vi "SetMaxDrivingPower.vi"(9 "Reinit":bool, 10 "HMI to Control":T1, 11 "SensorInputData":T2) -> (2 "HMI to ControlOut":T1, 3 "SensorInputDataOut":T2, 4 "Done":bool=TRUE)   [LabVIEW 2015]
uses:
  Gensubs/Maximum Power Allowed.vi
  Typedefs/SensorInputData.ctl
  Typedefs/HMI_to_Control.ctl
panel:
  in  "arguments":string[](array[string])
  in  "dt":i32
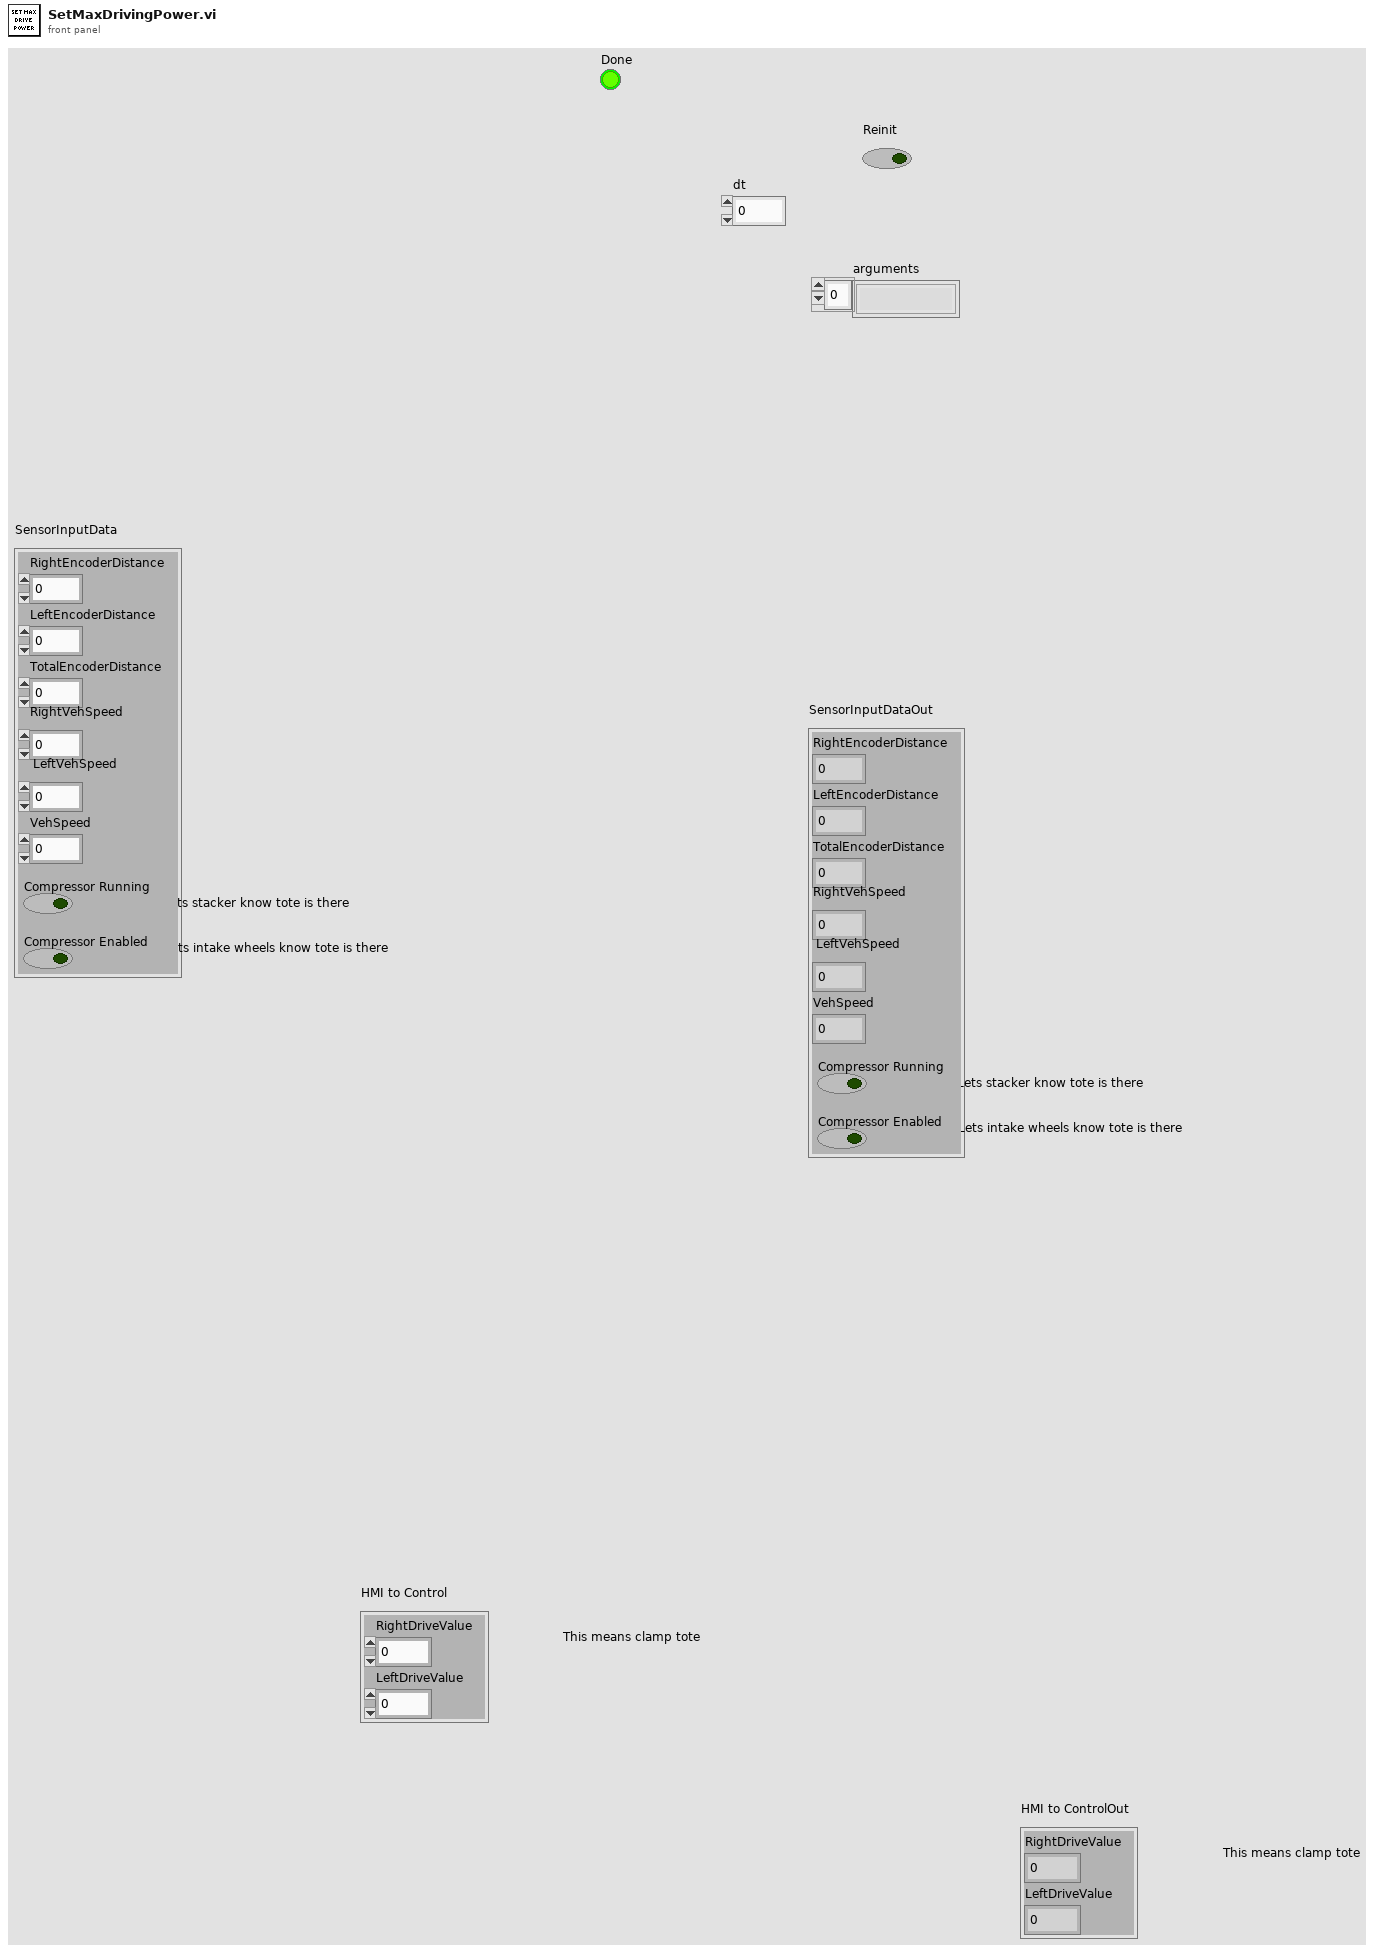
[diagram p1: front panel]
types:
  T1 = typedef "HMI_to_Control.ctl" = cluster{"RightDriveValue":dbl, "LeftDriveValue":dbl}
  T2 = typedef "SensorInputData.ctl" = cluster{"RightEncoderDistance":dbl, "LeftEncoderDistance":dbl, "TotalEncoderDistance":dbl, "RightVehSpeed":dbl, "LeftVehSpeed":dbl, "VehSpeed":dbl, "Compressor Running":bool, "Compressor Enabled":bool}
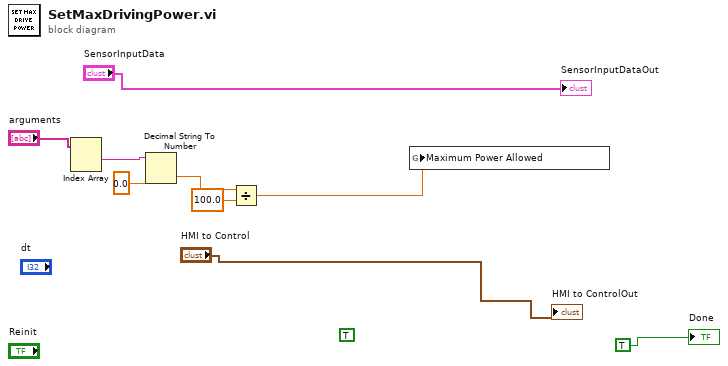
[diagram p0: block diagram]
diagram:
  (unwired) TRUE ("Inver. Wheels  In Request")
  n1 = Index Array(array="arguments") -> (element #1=w5:string)  [unwired: 2 in, 1 out]
  n2 = Decimal String To Number(string=w5, default (0L)=0.0) -> (number=w3:dbl)  [unwired: 1 in, 1 out]
  n3 = Divide(x=w3, y=100.0) -> (x/y=w1:dbl)
  n4 = global write "Maximum Power Allowed.vi" "Maximum Power Allowed"(w1) -> ()
  "SensorInputDataOut" <- "SensorInputData"
  "HMI to ControlOut" <- "HMI to Control"
  "Done" <- TRUE
